vi "Future.vi"(11 "Promise in":refnum<class "Promise.lvclass">) -> (2 "Future":refnum<class "Future.lvclass">, 3 "Promise":refnum<class "Promise.lvclass">)   [LabVIEW 2020, in "Promises.lvlib" / "Promise.lvclass"]
doc: "Retrieves the Future from the Promise that can be used to configure chaining (with <b>Then.vi</b>) and to retrieve the resolved result."
uses:
  Promise.lvclass
  Future/Future.lvclass
  Promise.lvclass/Promise.ctl
  Future/Future.lvclass/Future.ctl
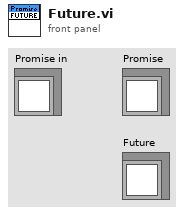
[diagram p1: front panel]
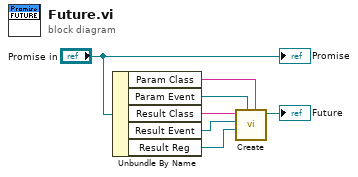
[diagram p0: block diagram]
diagram:
  n1 = Unbundle By Name("Promise in") -> ("Param Class"=w1:string, "Param Event"=w2:refnum<user-event>, "Result Class"=w6:string, "Result Event"=w5:refnum<user-event>, "Result Reg"=w4:refnum<event-registration>)
  n2 = call "Create.vi"("Param Class"=w1, "Param Event"=w2, "Result Reg"=w4, "Result Event"=w5, "Result Class"=w6) -> ("Future out"=→"Future":refnum<class "Future.lvclass">)  [unwired: 5 in, 1 out]
  "Promise" <- "Promise in"
